vi "ActionVIOnDownload.vi"(5 "System Definition Dir":path, 6 "IP address":string, 7 "Details Ref":refnum<vi>, 8 "error in (no error)":errorcluster, 10 "WebDAV session in":T1, 11 "Device Item Ref in":T2 format="%.0x") -> (0 "error out":errorcluster, 2 "WebDAV session out":T1, 3 "Device Item Ref out":T2 format="%.0x")   [LabVIEW 2019, in "HLA Custom Device System Explorer.lvlib"]
uses:
  HLA Custom Device System Explorer.lvlib
  <vilib>/NI VeriStand/Custom Device API/Custom Device Item Ref.ctl
  <vilib>/WebDAVClient/Advanced/SessionHandle.ctl
  <vilib>/NI VeriStand/Custom Device API/Custom Device API.lvlib
  <vilib>/WebDAVClient/NI_WebDAV.lvlib
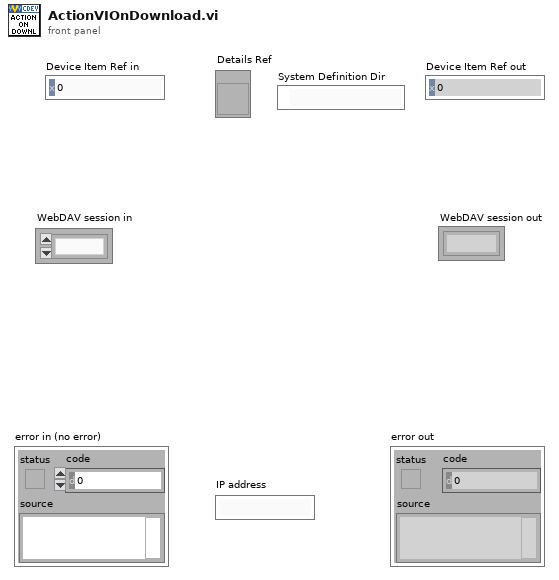
[diagram p1: front panel]
types:
  T1 = typedef "NI_WebDAV.lvlib/SessionHandle.ctl" = refnum<k1>
  T2 = typedef "Custom Device API.lvlib/Custom Device Item Ref.ctl" = u64
  T3 = typedef "HLA Custom Device Shared.lvlib/main_page_config.ctl" = cluster{"Federate Execution Name":string, "Federate Type":string, "Local Designator Settings":string, "FOM Module":path, "mak mtl file":path, "FOM destination path":string, "MTL destination path":string}
  T4 = typedef "Custom Device API.lvlib/Custom Device File Dependency.ctl" = cluster{"Source":T5, "RT Destination":path, "ForceDownload?":bool, "SupportedTarget":T7, "Version":string}
  T5 = typedef "Custom Device API.lvlib/Path Specification.ctl" = cluster{"Path":path, "Type":T6}
  T6 = typedef "Custom Device API.lvlib/Path Type.ctl" = enum16{"Absolute", "To Base", "To Common Data Dir", "To Application Data Dir"}
  T7 = typedef "Custom Device API.lvlib/Custom Device Supported Target.ctl" = enum16{"All", "PharLap", "VxWorks", "Windows", "Linux_32_ARM", "Linux_x64", "PharLap & Windows", "PharLap & VxWorks", "VxWorks & Windows"}
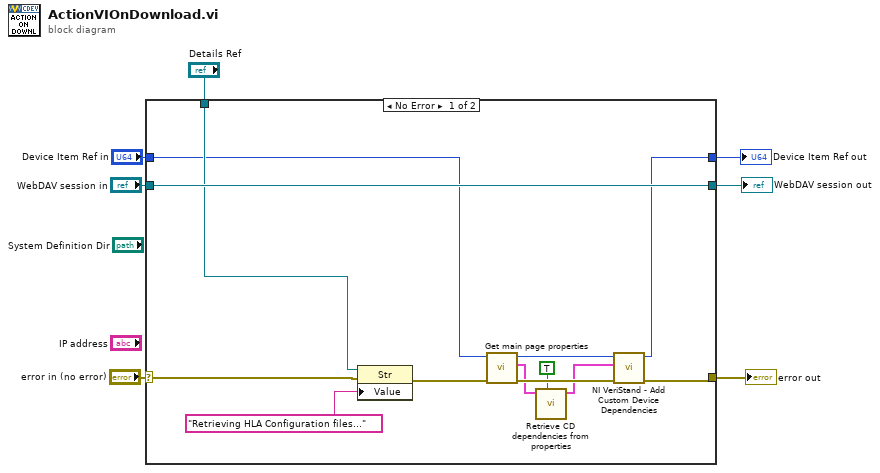
[diagram p0: block diagram]
diagram:
  n1 = case shown="No Error" "error in (no error)" {
    selector: "error in (no error)" -> [w10 w23]
    tunnel: [w11 w23] -> w6
    tunnel: "WebDAV session in" -> [w20 w22]
    tunnel: [w20 w22] -> w2
    tunnel: "Device Item Ref in" -> [w13 w21]
    tunnel: [w12 w21] -> w4
    tunnel: "Details Ref" -> [w19 _]
    frame No Error {
      n2 = property class="Str"(reference=w19, error in=w10, "Value"="Retrieving HLA Configuration files...") -> (error out=w9:errorcluster)  [unwired: 1 out]
      n3 = call "Get main page properties.vi"("error in"=w9, "Item Ref in"=w13) -> ("error out"=w16:errorcluster, "main page properties"=w15:T3, "Item Ref out"=w17:T2)  [unwired: 7 in]
      n4 = call "Retrieve CD dependencies from properties.vi"("ForceDownload?(F)"=TRUE, "main page properties in"=w15) -> ("custom device dependencies"=w8:T4[])  [unwired: 8 in, 1 out]
      n5 = call <vilib>:"NI VeriStand - Add Custom Device Dependencies.vi"("error in (no error)"=w16, "Dependencies"=w8, "Device Ref in"=w17) -> ("error out"=w11:errorcluster, "Device Ref out"=w12:T2)  [unwired: 7 in]
    }
    frame Error {
    }
  }
  "error out" <- w6
  "Device Item Ref out" <- w4
  "WebDAV session out" <- w2
